vi "Fdx Read (UDP-SAP).vi"(8 "error in":errorcluster, 10 "UdpHandle in":u32, 11 "InstrumentHandle_port in":u32) -> (0 "error out":errorcluster, 1 "Data":u8[](array[numeric])=[1, 2, 3, 4, 0, 0, 0, 0, 0, 0, 0, 0, 0, 0, 0, 0, 0, 0, 0, 0, 0, 0, 0, 0, 0, 0, 0, 0, 0, 0, 0, 0, 0, 0, 0, 0, 0, 0, 0, 0, 0, 0, 0, 0, 0, 0, 0, 0, 0, 0, 0, 0, 0, 0, 0, 0, 0, 0, 0, 0, 0, 0, 0, 0, 0, 0, 0, 0, 0, 0, 0, 0, 0, 0, 0, 0, 0, 0, 0, 0, 0, 0, 0, 0, 0, 0, 0, 0, 0, 0, 0, 0, 0, 0, 0, 0, 0, 0, 0, 0] format="%.0x", 2 "UdpHandle out":u32, 3 "InstrumentHandle_port out":u32, 4 "MsgRead":u32)   [LabVIEW 2020, in "AIM664LV.lvlib"]
uses:
  AIM664LV.lvlib
panel:
  in  "MsgCount(1)":u32=1
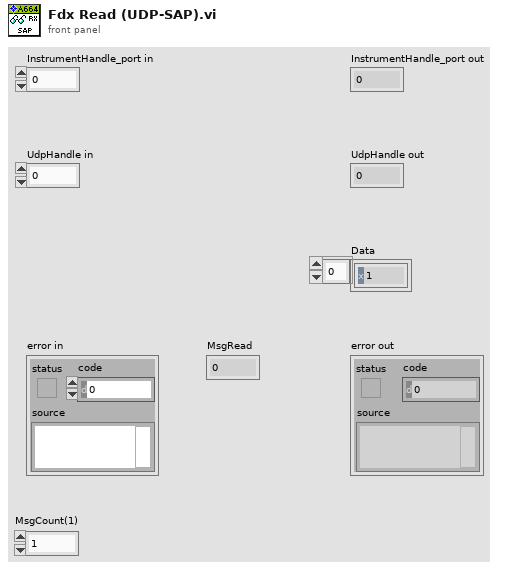
[diagram p1: front panel]
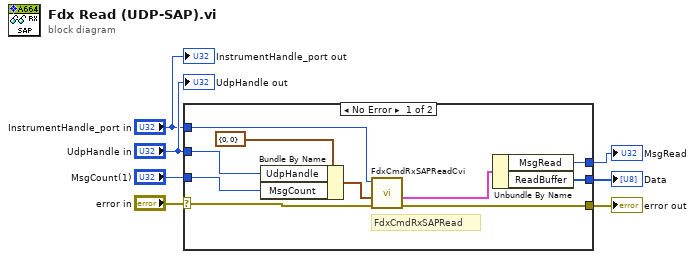
[diagram p0: block diagram]
diagram:
  n1 = case shown="No Error" "error in" {
    selector: "error in" -> [w17 w18]
    tunnel: [w14 w18] -> w6
    tunnel: "MsgCount(1)" -> [w13 _]
    tunnel: "UdpHandle in" -> [w12 _]
    tunnel: "InstrumentHandle_port in" -> [w11 _]
    tunnel: [w9 _] -> w1
    tunnel: [w8 _] -> w2
    frame No Error {
      # "FdxCmdRxSAPRead"
      n2 = Bundle By Name(cluster=cluster{"UdpHandle":u32, "MsgCount":u32} {"UdpHandle"=0, "MsgCount"=0} ("SapReadIn"), "UdpHandle"=w12, "MsgCount"=w13) -> (w16:cluster{"UdpHandle":u32, "MsgCount":u32})
      n3 = call "FdxCmdRxSAPReadCvi.vi"("error in"=w17, "SapReadIn"=w16, "InstrumentHandle_port"=w11) -> ("error out"=w14:errorcluster, "SapReadOut"=w10:cluster{"MsgRead":u32, "ReadBuffer":u8[]})  [unwired: 6 in, 1 out]
      n4 = Unbundle By Name(w10) -> ("MsgRead"=w9:u32, "ReadBuffer"=w8:u8[])
    }
    frame Error {
    }
  }
  "error out" <- w6
  "Data" <- w2
  "MsgRead" <- w1
  "UdpHandle out" <- "UdpHandle in"
  "InstrumentHandle_port out" <- "InstrumentHandle_port in"
